vi "Send Unregister Event.vi"(7 "Event":refnum<class "Event.lvclass">, 8 "Error In":errorcluster, 10 "Registrant Address":refnum<class "Message Enqueuer.lvclass">, 11 "Event Source Address":refnum<class "Message Enqueuer.lvclass">) -> (0 "Error Out":errorcluster, 3 "Event Source Address Out":refnum<class "Message Enqueuer.lvclass">)   [LabVIEW 2015, in "Event Source.lvlib" / "Unregister Event Msg.lvclass"]
doc: "Send an unregister event message to the Event Source Actor."
uses:
  Unregister Event Msg.lvclass
  <vilib>/ActorFramework/Message Enqueuer/Message Enqueuer.lvclass
  Event/Event.lvclass
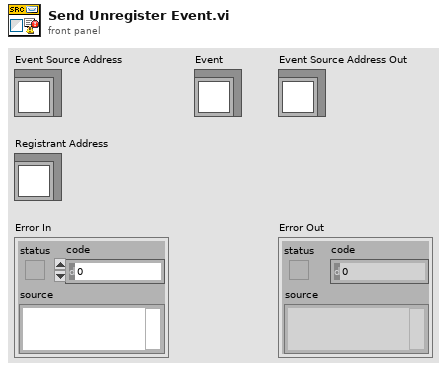
[diagram p1: front panel]
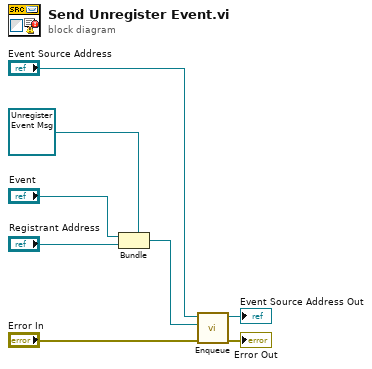
[diagram p0: block diagram]
diagram:
  n1 = Bundle(cluster=refnum<class "Unregister Event Msg.lvclass"> refnum ("Message Type"), "Event", "Registrant Address") -> (w4:refnum<class "Unregister Event Msg.lvclass">)
  n2 = call <vilib>:"Enqueue.vi"("error in (no error)"="Error In", "Message"=w4, "Message Enqueuer in"="Event Source Address") -> ("error out"=→"Error Out":errorcluster, "Message Enqueuer out"=→"Event Source Address Out":refnum<class "Message Enqueuer.lvclass">)  [unwired: 7 in]
